vi "Simple Test.vi"() -> ()   [LabVIEW 2018]
uses:
  Host-Control's/DTT Test folder Name's.ctl
  c5891c8d-faf9-4029-bd91-c8597a65e04f.vi
panel:
  out "Array 3":string[](array[string])
  out "Array 2":i32[](array[numeric])
  out "Array":string[](array[string])
  # "Voltage & currentt"
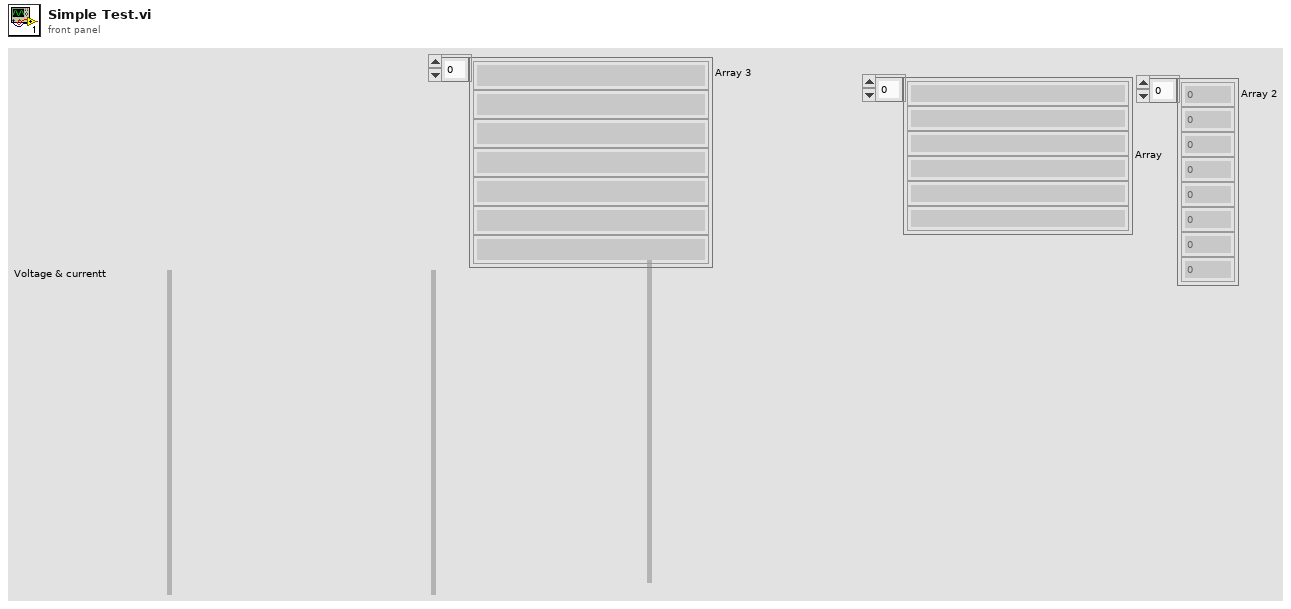
[diagram p1: front panel]
types:
  T1 = typedef "DTT Test folder Name's.ctl" = enum16{"Event Log", "Auto Sequence Configuration", "Channel Configuration's"}
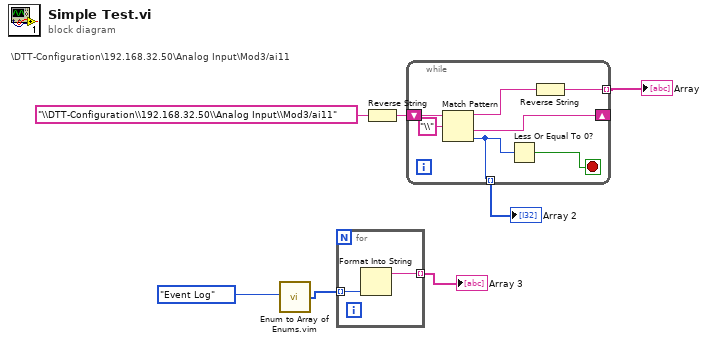
[diagram p0: block diagram]
diagram:
  # "\\DTT-Configuration\\192.168.32.50\\Analog Input\\Mod3/ai11"
  n1 = call "Enum to Array of Enums.vim"("enum"=DTT_Test_folder_Name's."Event Log" ("Folder Name")) -> ("array of enums"=w2:T1[])
  n2 = for {
    tunnel: [w9] -> w1 mode=indexing
    tunnel: w2 -> [w8] mode=indexing
    n3 = Format Into String(w8) -> (resulting string=w9:string)  [unwired: 3 in, 1 out]
  }
  "Array 3" <- w1
  n4 = Reverse String(1:"\\DTT-Configuration\\192.168.32.50\\Analog Input\\Mod3/ai11") -> (0:w6:string)
  n5 = while {
    shift-right: [w14] -> _
    shift-left: w6 -> [w15]
    tunnel: [w12] -> w5 mode=indexing
    tunnel: [w10] -> w4 mode=indexing
    stop <- w11 stop-if-true
    n6 = Match Pattern(string=w15, regular expression="\\") -> (before substring=w13:string, after substring=w14:string, offset past match=w10:i32)  [unwired: 1 in, 1 out]
    n7 = Less Or Equal To 0?(x=w10) -> (x <= 0?=w11:bool)
    n8 = Reverse String(1:w13) -> (0:w12:string)
  }
  "Array" <- w5
  "Array 2" <- w4
